vi "Convert I16 Data to SGL Data.vi"(4 "error in":errorcluster, 7 "refnum in":refnum<file>) -> (0 "error out":errorcluster, 3 "refnum out":refnum<file>)   [LabVIEW 2017]
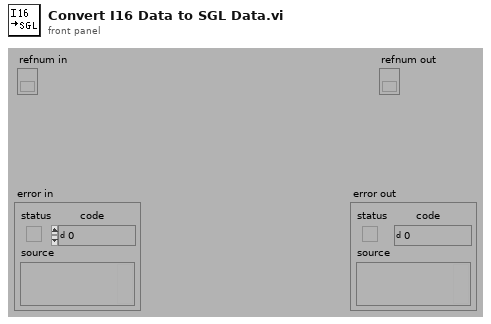
[diagram p1: front panel]
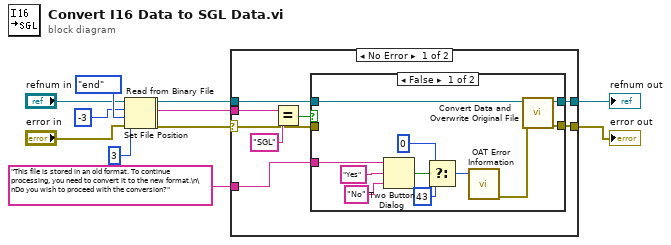
[diagram p0: block diagram]
diagram:
  n1 = Set File Position(offset (in bytes) (0)=-3 ("pos offset (0)"), refnum="refnum in", from (0:start)=enum16{"start", "end", "current"}."end" ("pos mode (0:2)"), error in="error in") -> (refnum out=w2:refnum<file>, error out=w1:errorcluster)
  n2 = Read from Binary File(8:w1, 10:3 ("count"), 11:w2) -> (0:w4:errorcluster, 2:w3:string, 3:w10:refnum<file>)  [unwired: 3 in, 1 out]
  n3 = case shown="No Error" w4 {
    selector: w4 -> [w14 w35]
    tunnel: w10 -> [w21 w36]
    tunnel: [w20 w36] -> w7
    tunnel: [w19 w35] -> w6
    tunnel: "This file is stored in an old format. To continue processing, you need to convert it to the new format.\n\nDo you wish to proceed with the conversion?" ("message") -> [w16 _]
    tunnel: w3 -> [w17 _]
    frame No Error {
      n4 = Equal?(x=w17, y="SGL") -> (x = y?=w15:bool)
      n5 = case shown="False" w15 {
        tunnel: w21 -> [w32 w33]
        tunnel: [w31 w33] -> w20
        tunnel: [w30 w34] -> w19
        tunnel: w16 -> [w27 _]
        tunnel: w14 -> [_ w34]
        frame False {
          n6 = Two Button Dialog(message=w27, 1:"No" ("F button name (\"Cancel\")"), 2:"Yes" ("T button name (\"OK\")")) -> (T button?=w26:bool)
          n7 = Select(t=0, s=w26, f=43 ("error code")) -> (s? t:f=w23:i32)
          n8 = call <vilib>:"OAT Error Information.vi"("error code"=w23) -> ("error out"=w22:errorcluster)  [unwired: 6 in]
          n9 = call <vilib>:"Convert Data and Overwrite Original File.vi"("error in"=w22, "refnum in"=w32) -> ("error out"=w30:errorcluster, "refnum out"=w31:refnum<file>)  [unwired: 8 in]
        }
        frame True {
        }
      }
    }
    frame Error {
    }
  }
  "refnum out" <- w7
  "error out" <- w6
